vi "Initialize.vi"(8 "error in (no error)":errorcluster, 10 "Peasant":T1, 11 "Peasant in":refnum<class "Peasant.lvclass">) -> (0 "error out":errorcluster, 3 "Peasant out":refnum<class "Peasant.lvclass">)   [LabVIEW 2021]
uses:
  Peasant.lvclass
  PeasantCluster.ctl
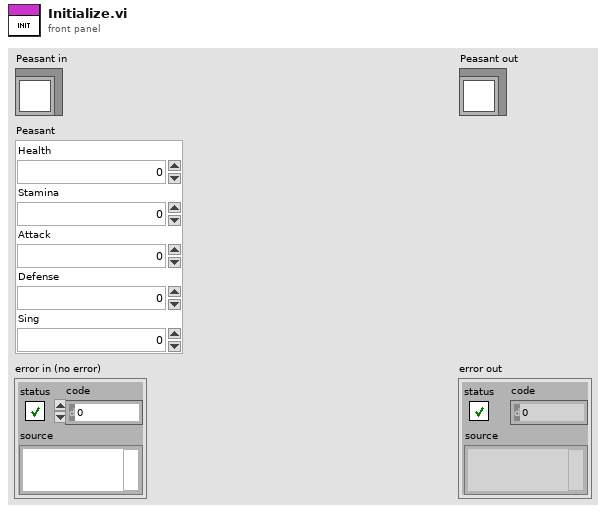
[diagram p1: front panel]
types:
  T1 = typedef "PeasantCluster.ctl" = cluster{"Health":i32, "Stamina":i32, "Attack":i32, "Defense":i32, "Sing":i32}
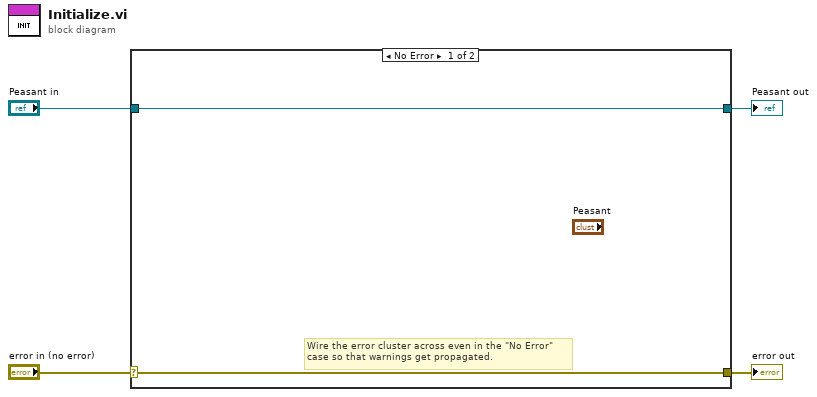
[diagram p0: block diagram]
diagram:
  n1 = case shown="No Error" "error in (no error)" {
    selector: "error in (no error)" -> [w5 w8]
    tunnel: [w5 w8] -> w3
    tunnel: [w6 w7] -> w1
    tunnel: "Peasant in" -> [w6 w7]
    frame No Error {
      # "Wire the error cluster across even in the \"No Error\"\ncase so that warnings get propagated."
    }
    frame Error {
    }
  }
  "error out" <- w3
  "Peasant out" <- w1
